vi "getCost.vi"(8 "error in (no error)":errorcluster, 11 "DarkRoast in":refnum<class "DarkRoast.lvclass">) -> (0 "error out":errorcluster, 2 "cost":dbl, 3 "DarkRoast out":refnum<class "DarkRoast.lvclass">)   [LabVIEW 2018, in "DarkRoast.lvclass"]
uses:
  DarkRoast.lvclass
  Beverage Class/Beverage.lvclass
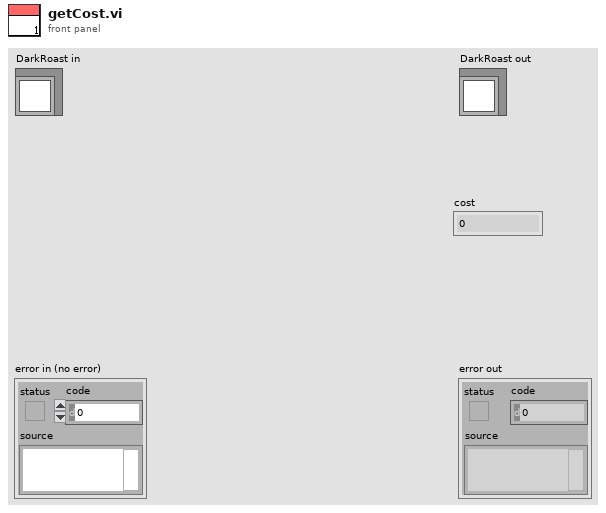
[diagram p1: front panel]
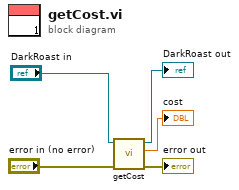
[diagram p0: block diagram]
diagram:
  n1 = call-parent "getCost.vi"("error in (no error)"="error in (no error)", "Beverage in"="DarkRoast in") -> ("error out"=→"error out":errorcluster, "cost"=→"cost":dbl, "Beverage out"=→"DarkRoast out":refnum<class "DarkRoast.lvclass">)  [unwired: 7 in]
